vi "Spectrometer_R&S_2017.04.10.vi"(11 "position_xyz":T2 {"Position Z" min=0.0 max=10.0 step=0.001 format="%.3f"; "Position Y" min=-10.0 max=10.0 step=0.1 format="%.3f"; "Position X" min=-10.0 max=10.0 step=0.1 format="%.3f"}) -> ()   [LabVIEW 2014]
uses:
  <vilib>/DAQmx/write.llb/DAQmx Write (Digital Bool 1Line 1Point).vi
  <vilib>/Analysis/baseanly.llb/Vector x A.vi
  GLOBAL_VAR.vi
  <vilib>/DAQmx/miscellaneous.llb/DAQmx Fill In Error Info.vi
  <vilib>/Analysis/Matrix/Numeric/Conversions/Array To Matrix - RA2.vi
  <vilib>/DAQmx/create/channels.llb/DAQmx Create Channel (CO-Pulse Generation-Ticks).vi
  <vilib>/DAQmx/create/channels.llb/DAQmx Create Channel (DO-Digital Output).vi
  <vilib>/DAQmx/configure/trigger.llb/DAQmx Start Trigger (Digital Edge).vi
  <resource>/objmgr/daqmx.rc
  <vilib>/Analysis/NI_AALBase.lvlib
  <vilib>/Analysis/Matrix/NI_Matrix.lvlib
  <instrlib>/Rohde&Schwarz RF Signal Generator/Rohde&Schwarz RF Signal Generator.lvlib
panel:
  in  "sweep_parameters":T1={"Repetitions"=1, "Power dBm"=5.999999061226845, "Freq Start [Hz]"=2800000000.0, "Freq Stop [Hz]"=3000000000.0, "Step size [Hz]"=2500000.0, "Dwell Time [ms]"=0.09999999974525053} {"Dwell Time [ms]" format="%.3f"; "Step size [Hz]" format="%.2p"; "Freq Stop [Hz]" format="%.2p"; "Freq Start [Hz]" format="%.2p"; "Power dBm" format="%.2f"; "Repetitions" min=1 max=1000 step=1}
  out "File name":string
  in  "Save":bool
  in  "Stop":bool
  in  "generator_enable":bool
  out "Run":i32=100
  out "Remain":i32
  out "Intensity Graph":ext[][](graph)
  out "Histogram":cluster{ext[], ext[]}[](graph)=[{[2700000000.0, 2702500000.0, 2705000000.0, 2707500000.0, 2710000000.0, 2712500000.0, 2715000000.0, 2717500000.0, 2720000000.0, 2722500000.0, 2725000000.0, 2727500000.0, 2730000000.0, 2732500000.0, 2735000000.0, 2737500000.0, 2740000000.0, 2742500000.0, 2745000000.0, 2747500000.0, 2750000000.0, 2752500000.0, 2755000000.0, 2757500000.0, 2760000000.0, 2762500000.0, 2765000000.0, 2767500000.0, 2770000000.0, 2772500000.0, 2775000000.0, 2777500000.0, 2780000000.0, 2782500000.0, 2785000000.0, 2787500000.0, 2790000000.0, 2792500000.0, 2795000000.0, 2797500000.0, 2800000000.0, 2802500000.0, 2805000000.0, 2807500000.0, 2810000000.0, 2812500000.0, 2815000000.0, 2817500000.0, 2820000000.0, 2822500000.0, 2825000000.0, 2827500000.0, 2830000000.0, 2832500000.0, 2835000000.0, 2837500000.0, 2840000000.0, 2842500000.0, 2845000000.0, 2847500000.0, 2850000000.0, 2852500000.0, 2855000000.0, 2857500000.0, 2860000000.0, 2862500000.0, 2865000000.0, 2867500000.0, 2870000000.0, 2872500000.0, 2875000000.0, 2877500000.0, 2880000000.0, 2882500000.0, 2885000000.0, 2887500000.0, 2890000000.0, 2892500000.0, 2895000000.0, 2897500000.0, 2900000000.0, 2902500000.0, 2905000000.0, 2907500000.0, 2910000000.0, 2912500000.0, 2915000000.0, 2917500000.0, 2920000000.0, 2922500000.0, 2925000000.0, 2927500000.0, 2930000000.0, 2932500000.0, 2935000000.0, 2937500000.0, 2940000000.0, 2942500000.0, 2945000000.0, 2947500000.0, 2950000000.0, 2952500000.0, 2955000000.0, 2957500000.0, 2960000000.0, 2962500000.0, 2965000000.0, 2967500000.0, 2970000000.0, 2972500000.0, 2975000000.0, 2977500000.0, 2980000000.0, 2982500000.0, 2985000000.0, 2987500000.0, 2990000000.0, 2992500000.0, 2995000000.0, 2997500000.0, 3000000000.0], [26841.121559672197128, 27464.174520667373477, 27576.32405364650522, 29408.099758972323686, 27638.629349746022854, 27576.32405364650522, 27638.629349746022854, 27651.09040896592638, 28398.753962160138, 28311.526547620813311, 28236.76019230139215, 27912.772652583900449, 27850.467356484382814, 27875.389474924189868, 28174.454896201874515, 28697.819383437822648, 28685.35832421791912, 28535.825613579076798, 28809.968916416954391, 29046.729041595121403, 28647.975146558208541, 28523.36455435917327, 28062.305363222742772, 28174.454896201874515, 28473.520317479559163, 27738.31782350525107, 28423.676080599945054, 29133.956456134446093, 28859.8131532965685, 27638.629349746022854, 29133.956456134446093, 27763.239941945058124, 27352.024987688241733, 27439.252402227566423, 28822.429975636857918, 27526.479816766891112, 28548.286672798980325, 27838.006297264479286, 28847.352094076664972, 28884.735271736375553, 29271.02810755338489, 28884.735271736375553, 27289.7196915887241, 28971.962686275700243, 28336.448666060620365, 28548.286672798980325, 27975.077948683418082, 27763.239941945058124, 29470.405055071841321, 28822.429975636857918, 28087.227481662549826, 28286.604429181006259, 27352.024987688241733, 27401.869224567855841, 28398.753962160138, 29308.411285213095471, 28485.98137669946269, 28585.669850458690906, 28710.280442657726175, 28236.76019230139215, 28311.526547620813311, 27576.32405364650522, 27302.180750808627625, 28299.065488400909786, 26878.504737331907709, 28809.968916416954391, 29420.560818192227213, 28859.8131532965685, 27750.778882725154597, 28535.825613579076798, 28398.753962160138, 28261.682310741199204, 28947.040567835893189, 28361.370784500427419, 28785.046797977147337, 28610.59196889849796, 27476.635579887277004, 28062.305363222742772, 28311.526547620813311, 28809.968916416954391, 28647.975146558208541, 28112.14960010235688, 28822.429975636857918, 27738.31782350525107, 28199.377014641681569, 28510.903495139269744, 27451.71346144746995, 28074.766422442646299, 27725.856764285347543, 28635.514087338305014, 28834.891034856761445, 27376.947106128048787, 29096.573278474735512, 28274.143369961102731, 29034.267982375217876, 28560.747732018883852, 27277.258632368820573, 28884.735271736375553, 28049.844304002839245, 27975.077948683418082, 26965.732151871232396, 28809.968916416954391, 28000.000067123225136, 27127.725921729978248, 28037.383244782935718, 28000.000067123225136, 27277.258632368820573, 27800.623119604768705, 28087.227481662549826, 27501.557698327084058, 26778.816263572679492, 26429.906605415380737, 27526.479816766891112, 26442.367664635284264, 26479.750842294994845, 27775.701001164961651, 27040.498507190653559, 26429.906605415380737, 27750.778882725154597, 27464.174520667373477, 27925.233711803803976]}, {[2700000000.0, 2702500000.0, 2705000000.0, 2707500000.0, 2710000000.0, 2712500000.0, 2715000000.0, 2717500000.0, 2720000000.0, 2722500000.0, 2725000000.0, 2727500000.0, 2730000000.0, 2732500000.0, 2735000000.0, 2737500000.0, 2740000000.0, 2742500000.0, 2745000000.0, 2747500000.0, 2750000000.0, 2752500000.0, 2755000000.0, 2757500000.0, 2760000000.0, 2762500000.0, 2765000000.0, 2767500000.0, 2770000000.0, 2772500000.0, 2775000000.0, 2777500000.0, 2780000000.0, 2782500000.0, 2785000000.0, 2787500000.0, 2790000000.0, 2792500000.0, 2795000000.0, 2797500000.0, 2800000000.0, 2802500000.0, 2805000000.0, 2807500000.0, 2810000000.0, 2812500000.0, 2815000000.0, 2817500000.0, 2820000000.0, 2822500000.0, 2825000000.0, 2827500000.0, 2830000000.0, 2832500000.0, 2835000000.0, 2837500000.0, 2840000000.0, 2842500000.0, 2845000000.0, 2847500000.0, 2850000000.0, 2852500000.0, 2855000000.0, 2857500000.0, 2860000000.0, 2862500000.0, 2865000000.0, 2867500000.0, 2870000000.0, 2872500000.0, 2875000000.0, 2877500000.0, 2880000000.0, 2882500000.0, 2885000000.0, 2887500000.0, 2890000000.0, 2892500000.0, 2895000000.0, 2897500000.0, 2900000000.0, 2902500000.0, 2905000000.0, 2907500000.0, 2910000000.0, 2912500000.0, 2915000000.0, 2917500000.0, 2920000000.0, 2922500000.0, 2925000000.0, 2927500000.0, 2930000000.0, 2932500000.0, 2935000000.0, 2937500000.0, 2940000000.0, 2942500000.0, 2945000000.0, 2947500000.0, 2950000000.0, 2952500000.0, 2955000000.0, 2957500000.0, 2960000000.0, 2962500000.0, 2965000000.0, 2967500000.0, 2970000000.0, 2972500000.0, 2975000000.0, 2977500000.0, 2980000000.0, 2982500000.0, 2985000000.0, 2987500000.0, 2990000000.0, 2992500000.0, 2995000000.0, 2997500000.0, 3000000000.0], [27662.305362263847, 27614.704116043806, 27558.75396014644, 27479.62623410005, 27635.264863756656, 27635.514084941045, 27523.73838373851, 27614.704116043802, 27583.17763621744, 27571.58885114293, 27593.520315369973, 27605.109100444486, 27505.545237277456, 27540.685424277577, 27573.831841802512, 27521.74461426332, 27747.788228512374, 27553.395704681883, 27408.099754177805, 27507.040564383846, 27553.769536458476, 27450.09352374888, 27547.16517507192, 27590.529661157172, 27485.98137430221, 27331.838071751987, 27460.06237112481, 27420.436202805507, 27402.99071989765, 27434.64181031619, 27576.697885423117, 27476.38635870286, 27470.654271461714, 27460.311592309215, 27451.962682631867, 27448.722807234688, 27469.781997316335, 27462.056140599987, 27364.23682572375, 27414.081062603364, 27456.573274543232, 27499.688539444087, 27488.598196738385, 27439.252402227583, 27451.215019078678, 27574.45489476352, 27513.894146954794, 27562.741499096825, 27559.377013107456, 27384.42374165998, 27576.074832462113, 27480.747729429848, 27504.423741947663, 27448.099754273695, 27508.90972326683, 27439.50162341197, 27397.383243248685, 27424.54835234809, 27331.21501879102, 27477.258632848276, 27459.68853934821, 27434.267978539607, 27381.05925567063, 27417.07171681613, 27347.912838145676, 27456.82249572762, 27392.398819560723, 27427.539006560855, 27402.86610930546, 27384.79757343659, 27482.86610949723, 27504.049910171063, 27508.037449121424, 27430.778881958024, 27495.202558124915, 27442.367667032533, 27426.16829004667, 27367.60131171313, 27402.616888121054, 27600.00006616432, 27539.68853953999, 27533.58262052224, 27462.305361784383, 27564.361436795392, 27572.087293511737, 27503.55146780227, 27476.137137518494, 27474.766421004293, 27580.560813781274, 27579.813150228085, 27592.024988263576, 27505.296016093063, 27570.84118758975, 27614.953337228195, 27611.215019462234, 27484.236826011424, 27503.925299578863, 27544.54835263575, 27602.616888600503, 27550.903492837893, 27593.769536554377, 27516.63557998317, 27611.962683015438, 27551.028103430108, 27655.701000877292, 27659.688539827646, 27578.5670443061, 27729.59508205134, 27610.093524132444, 27489.968913252564, 27615.202558412602, 27486.479816671, 27421.059255766515, 27418.56704392252, 27449.221249603488, 27600.996950901917, 27543.92529967475, 27425.17140530909, 27466.04367955036, 27523.987604922913, 27501.183866550484]}]
  in  "start":bool
  in  "stop":bool
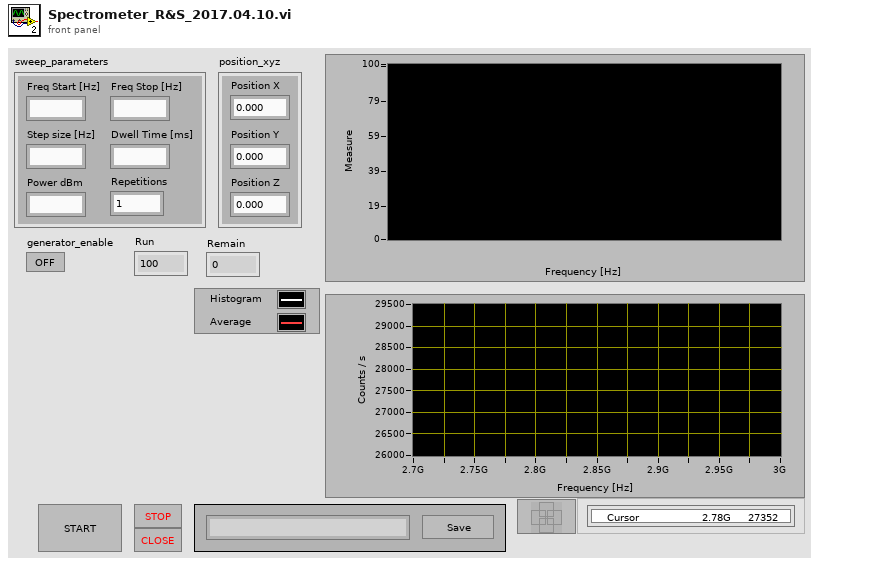
[diagram p1: front panel]
types:
  T1 = cluster{"Repetitions":i32, "Power dBm":ext, "Freq Start [Hz]":ext, "Freq Stop [Hz]":ext, "Step size [Hz]":ext, "Dwell Time [ms]":ext}
  T2 = cluster{"Position X":dbl, "Position Y":dbl, "Position Z":dbl}
  T3 = enum16{"stand-by", "init", "config", "acquisition", "processing", "close", "Set Variables"}
  T4 = typedef "NI_Matrix.lvlib/RealMatrix.ctl" = dbl[][]
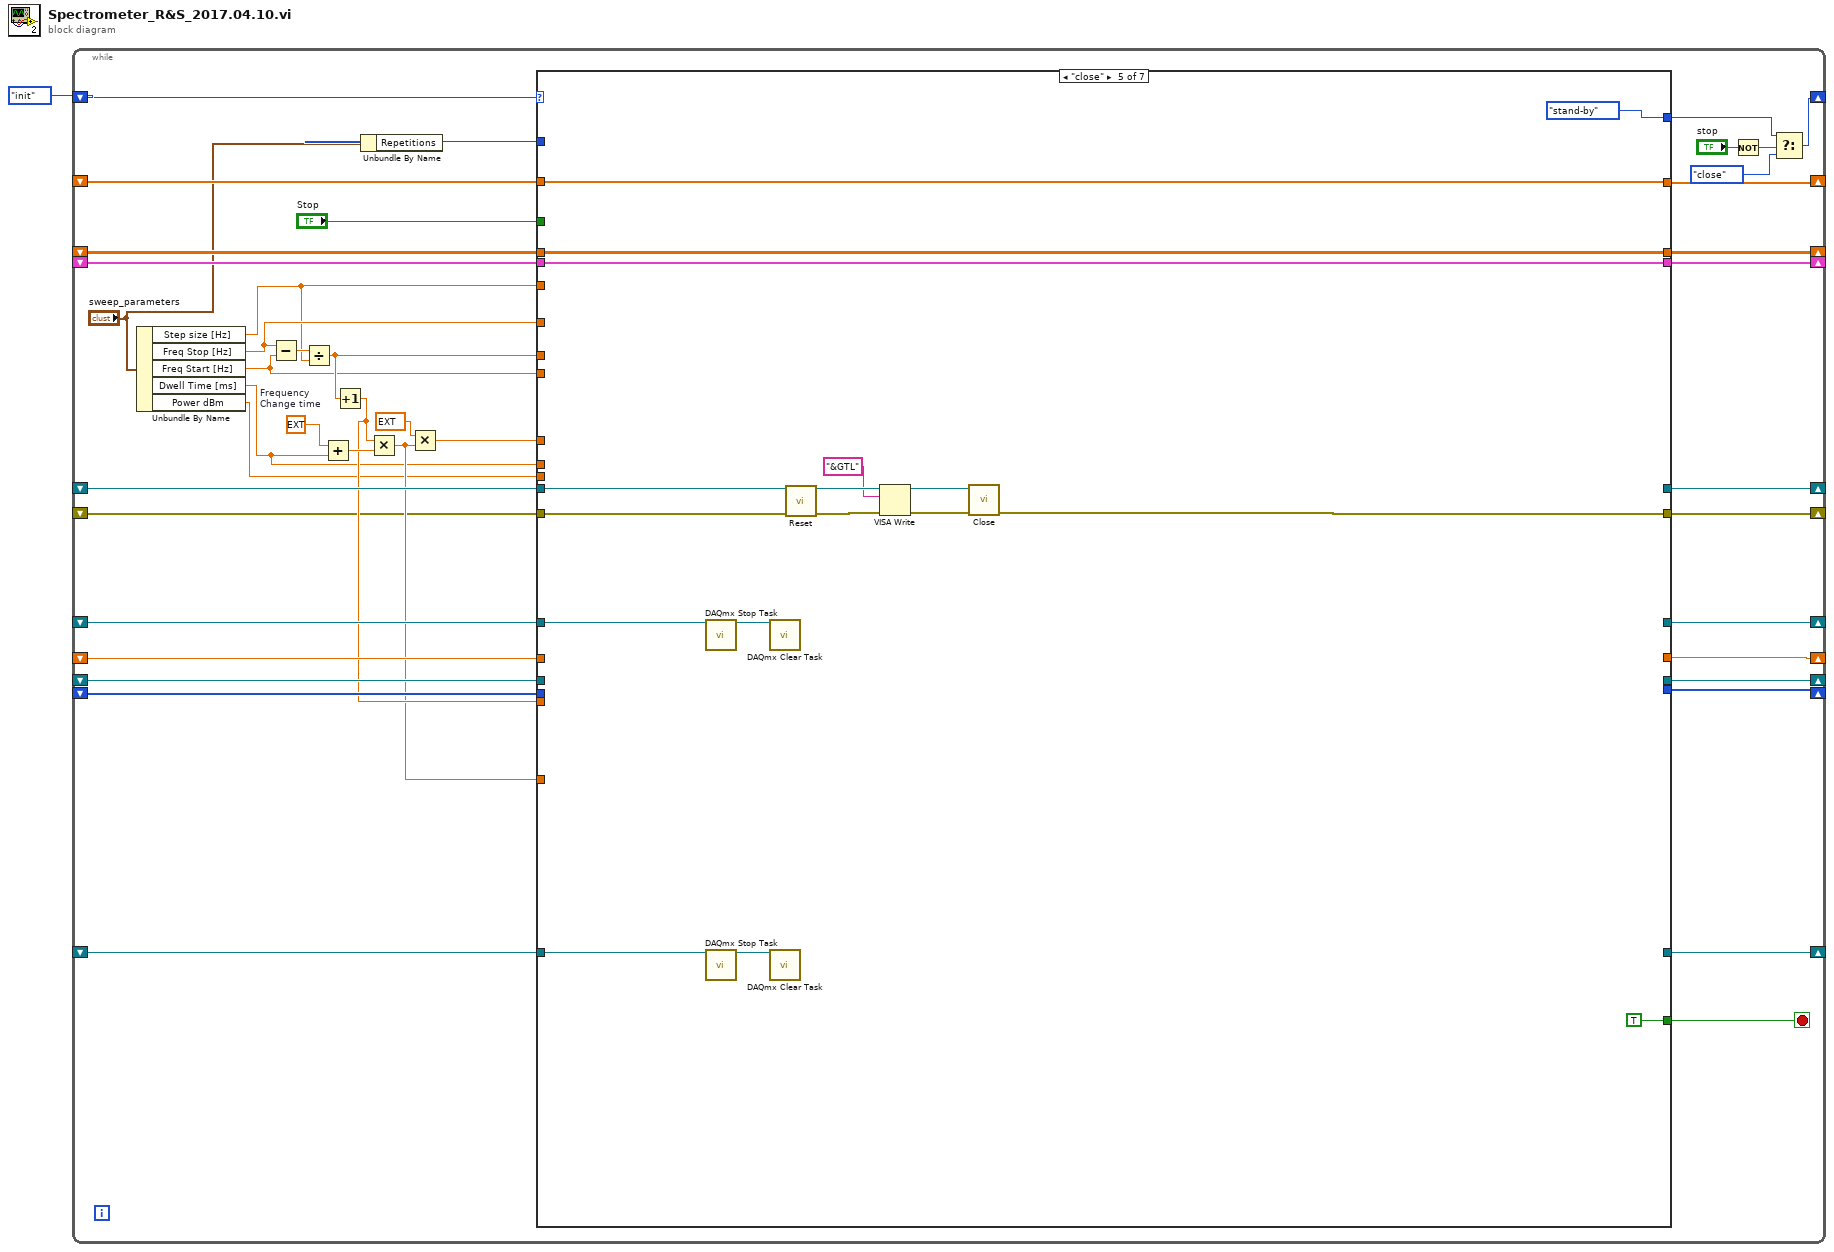
[diagram p0: block diagram]
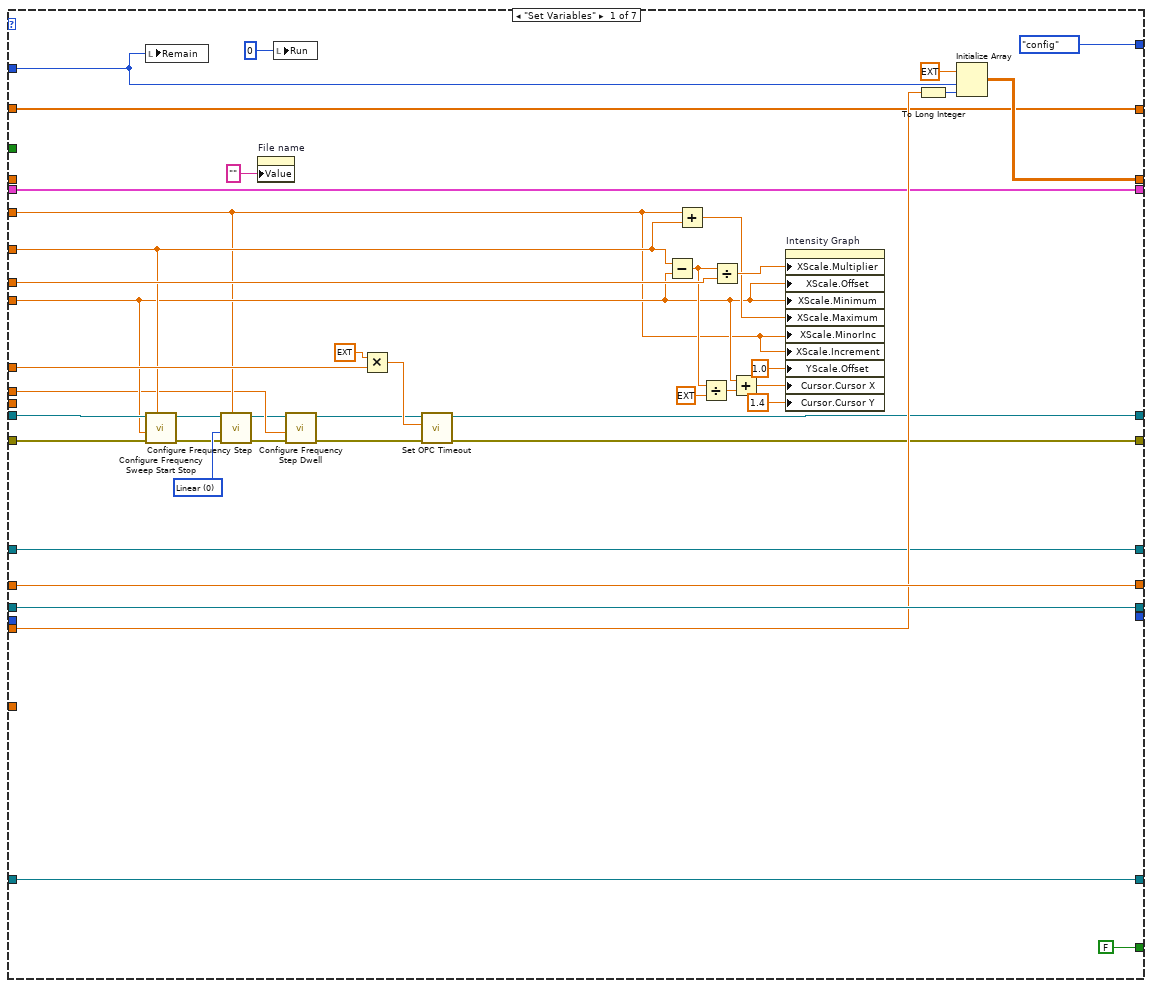
[diagram p2: hidden frame]
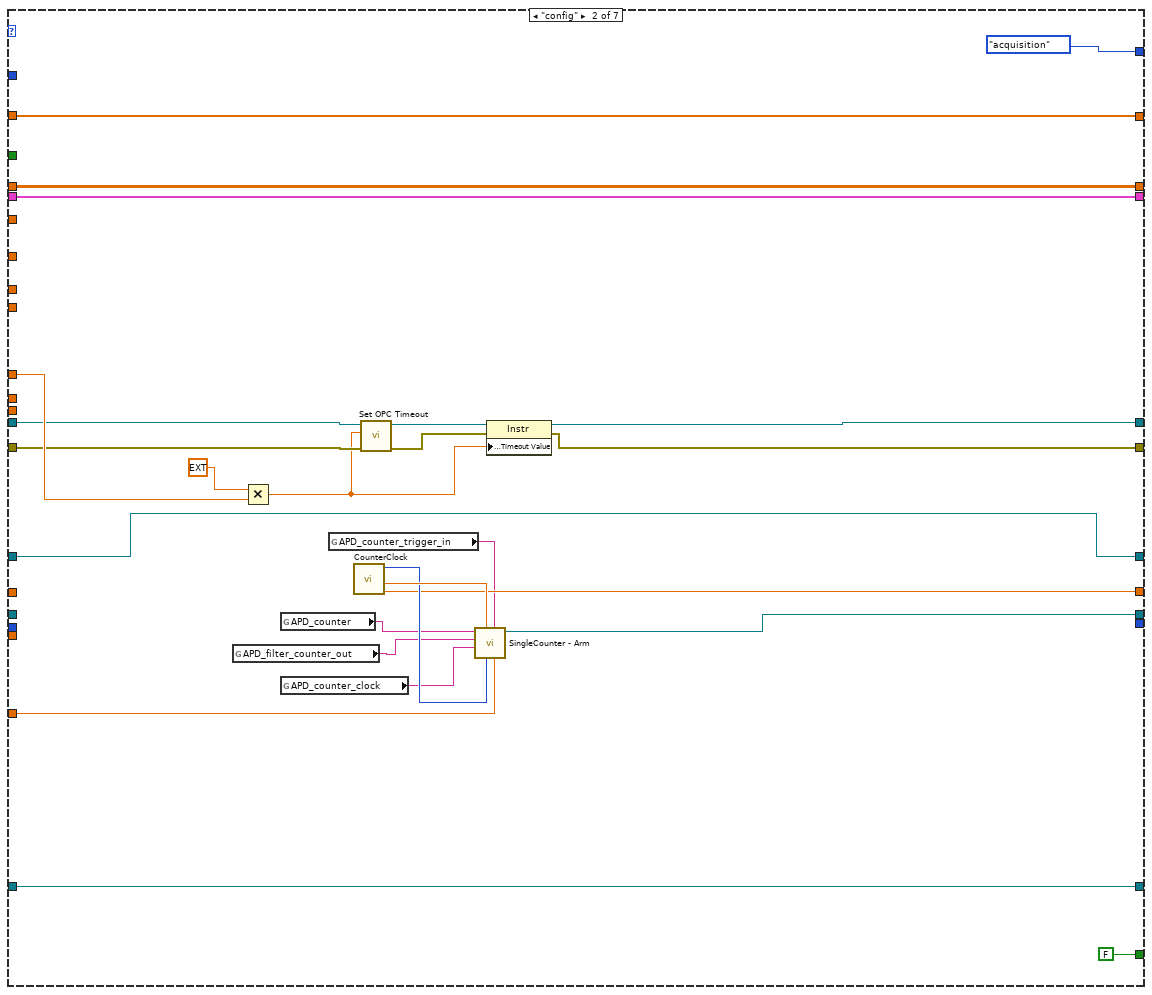
[diagram p3: hidden frame]
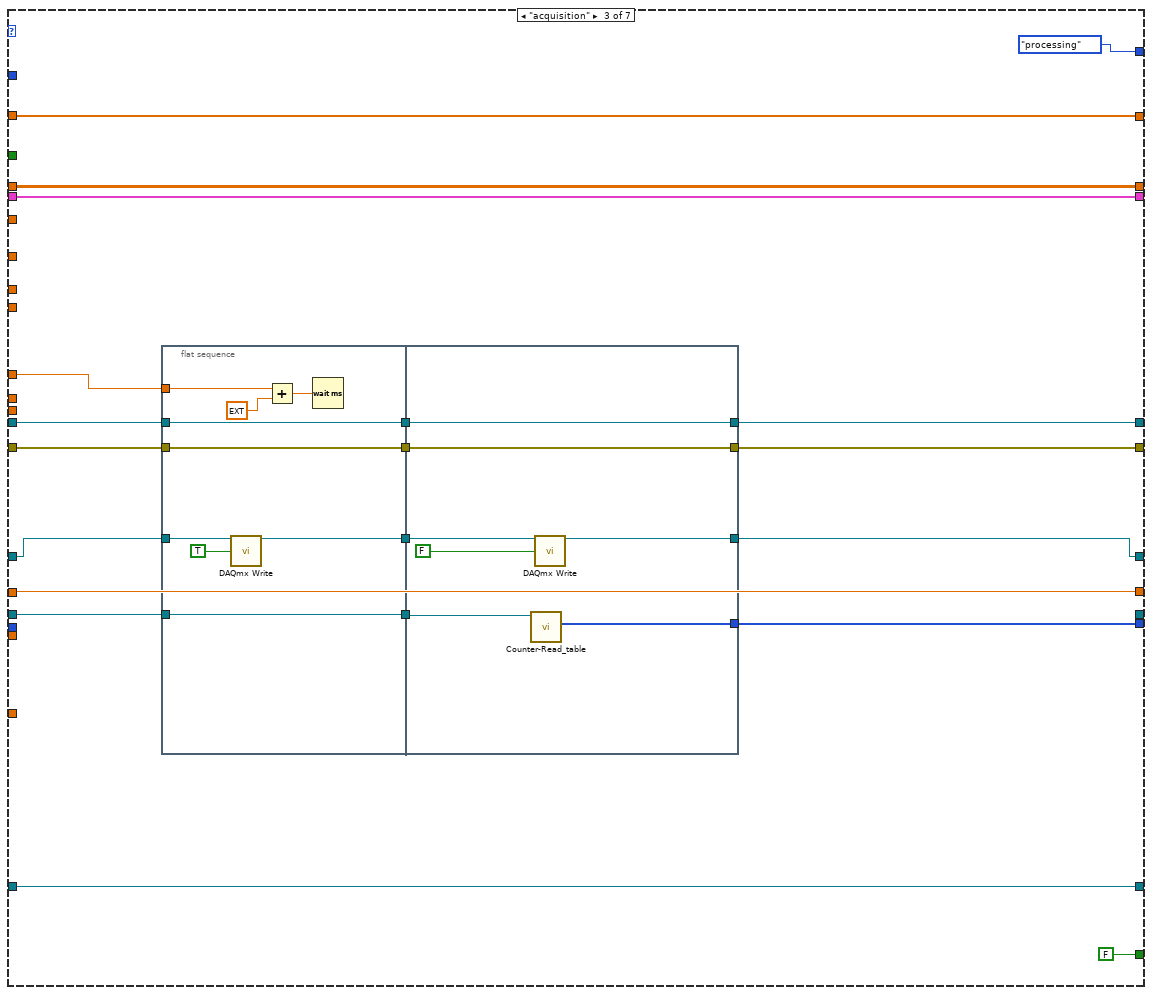
[diagram p4: hidden frame]
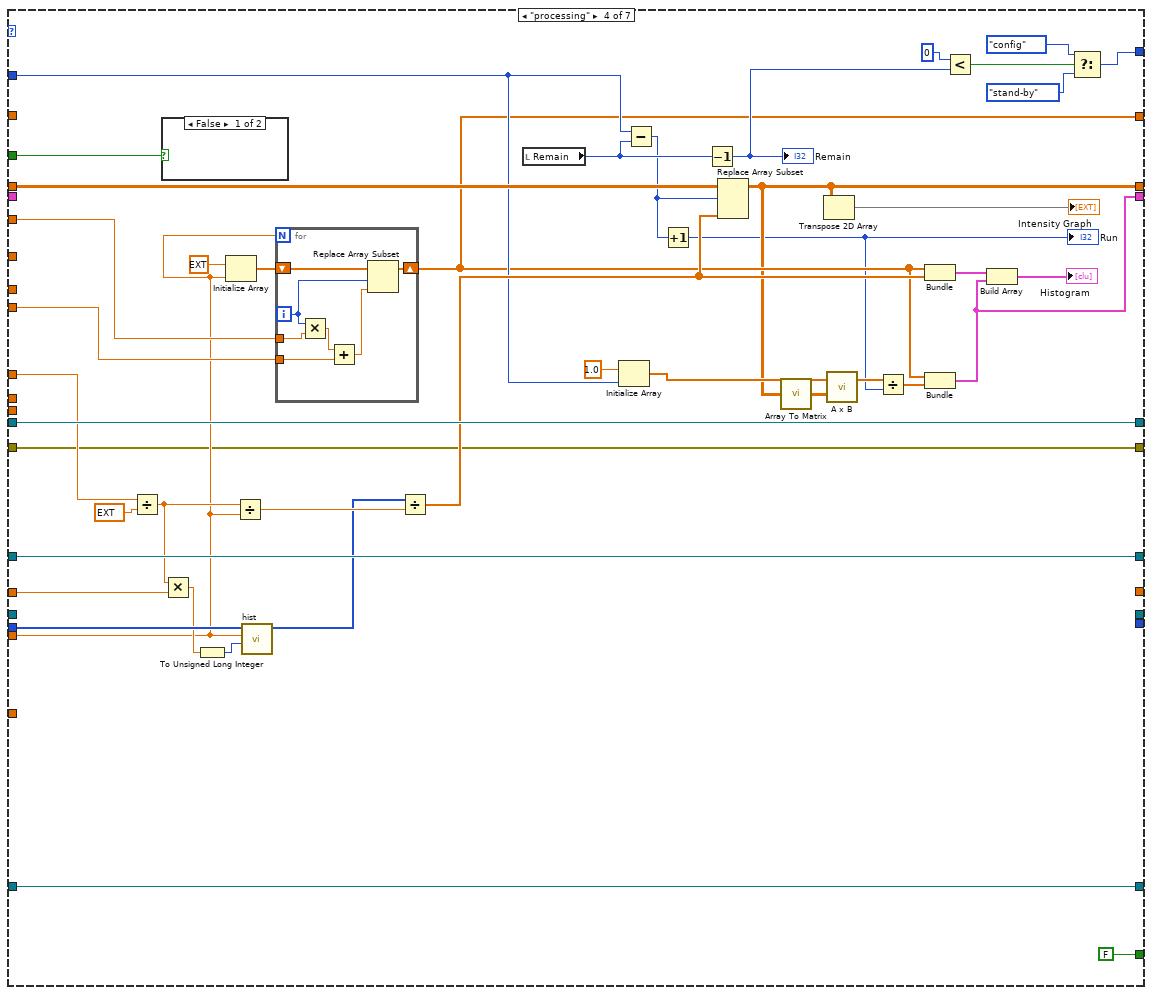
[diagram p5: hidden frame]
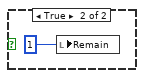
[diagram p6: hidden frame]
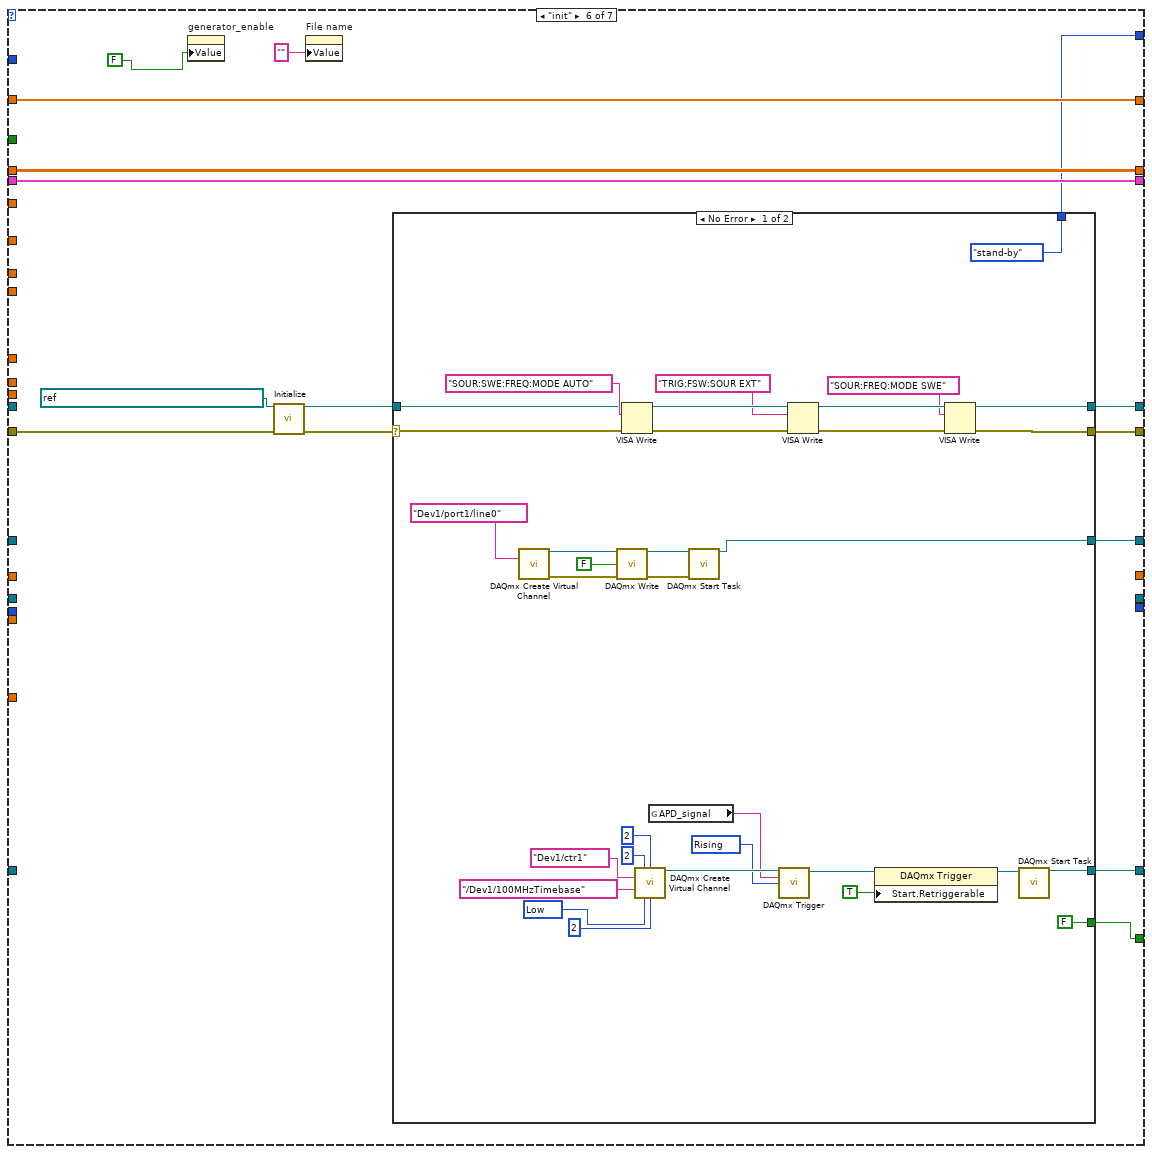
[diagram p7: hidden frame]
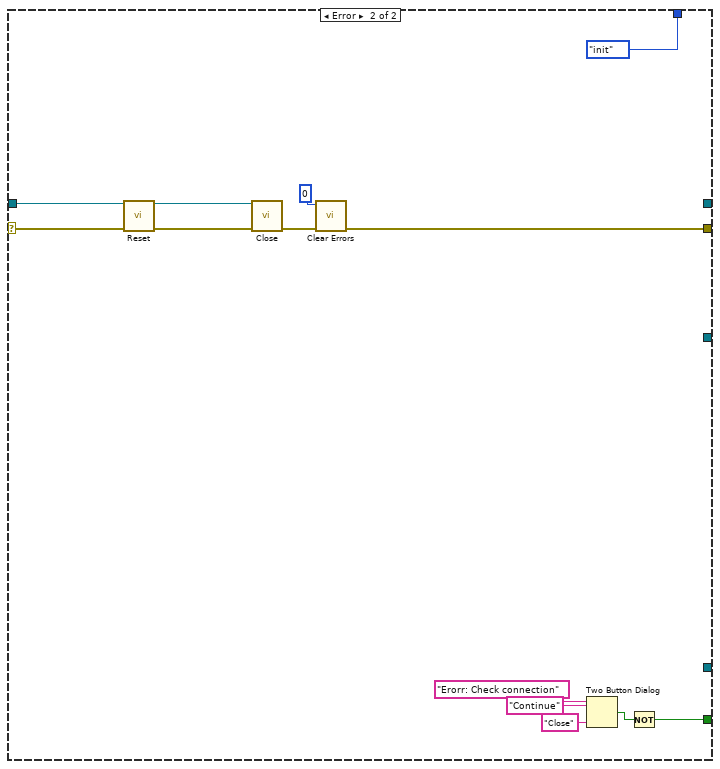
[diagram p8: hidden frame]
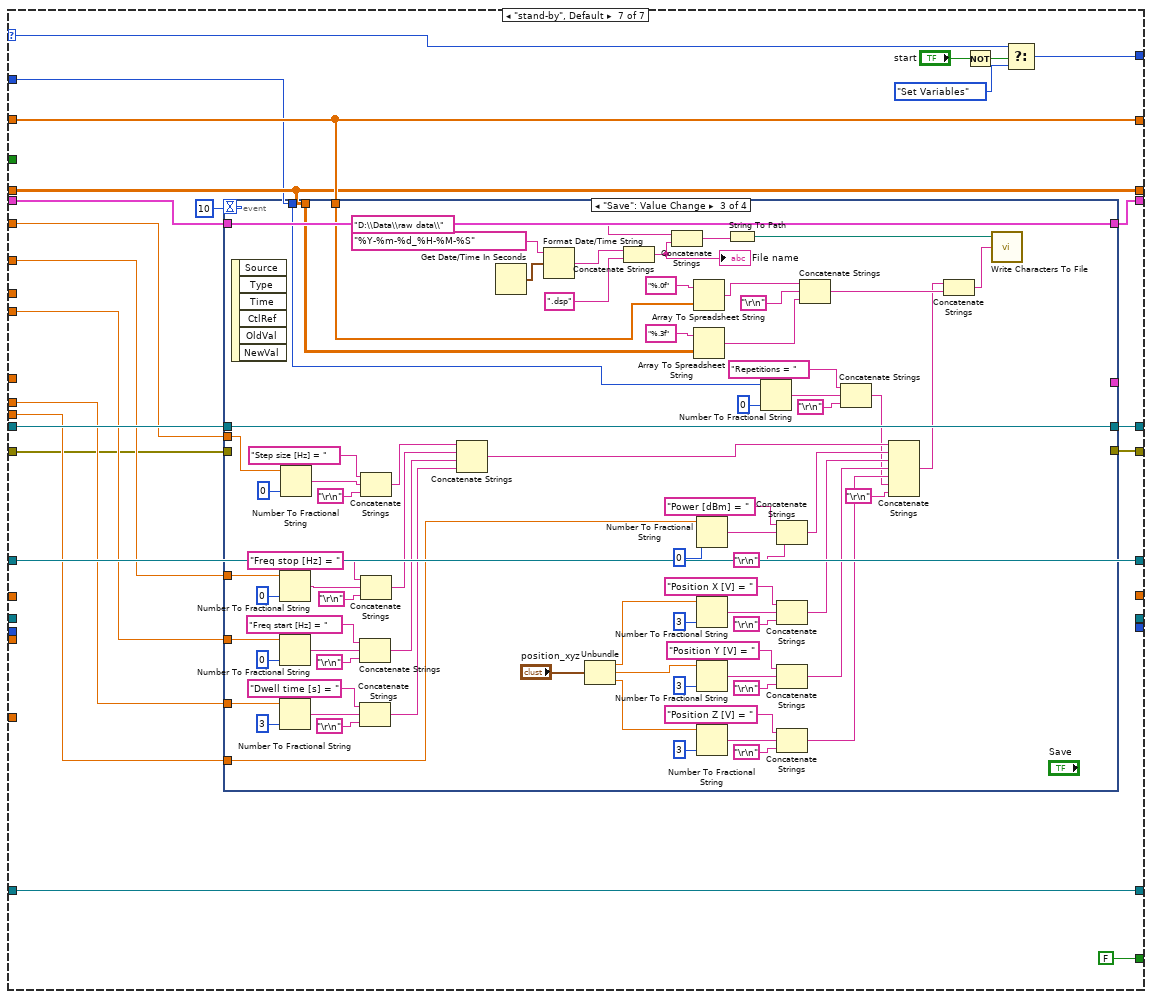
[diagram p9: hidden frame]
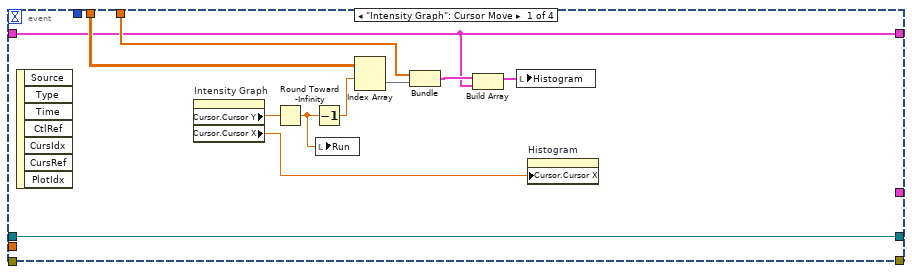
[diagram p10: hidden frame]
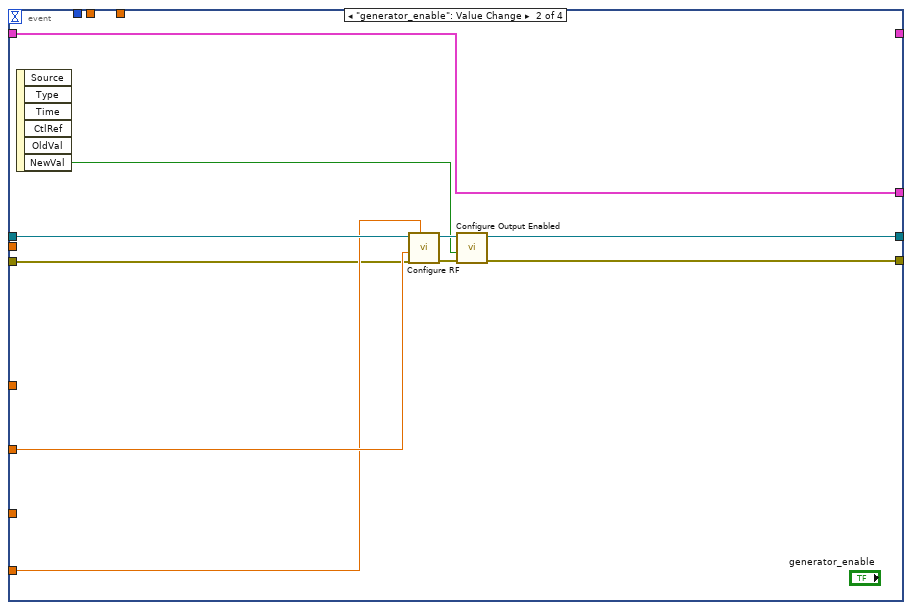
[diagram p11: hidden frame]
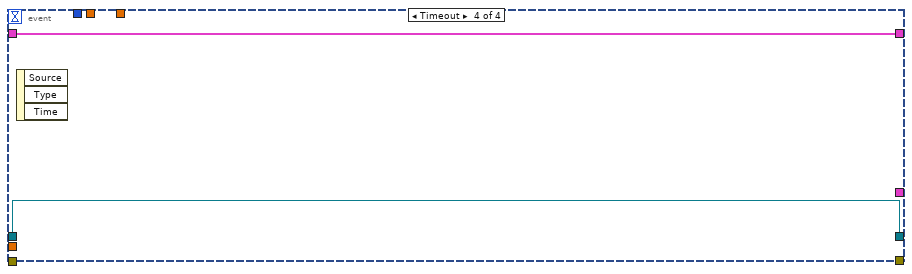
[diagram p12: hidden frame]
diagram:
  n1 = while {
    shift-right: [w30] -> _
    shift-left: T3."init" -> [w44]
    shift-right: [w40] -> _
    shift-left: _ -> [w39]
    shift-right: [w12] -> _
    shift-left: _ -> [w38]
    shift-right: [w37] -> _
    shift-left: _ -> [w36]
    shift-right: [w35] -> _
    shift-left: _ -> [w34]
    shift-right: [w28] -> _
    shift-left: _ -> [w27]
    shift-right: [w21] -> _
    shift-left: _ -> [w23]
    shift-right: [w20] -> _
    shift-left: _ -> [w19]
    shift-right: [w17] -> _
    shift-left: _ -> [w16]
    shift-right: [w15] -> _
    shift-left: _ -> [w14]
    shift-right: [w11] -> _
    shift-left: _ -> [w10]
    stop <- w29 stop-if-true
    w9 = ext 0.0  # Frequency Change time
    n2 = Unbundle By Name("sweep_parameters") -> ("Step size [Hz]"=w4:ext, "Freq Stop [Hz]"=w5:ext, "Freq Start [Hz]"=w3:ext, "Dwell Time [ms]"=w6:ext, "Power dBm"=w7:ext)
    n3 = Subtract(x=w5, y=w3) -> (x-y=w43:ext)
    n4 = Divide(x=w43, y=w4) -> (x/y=w24:ext)
    n5 = Add(x=w9, y=w6) -> (x+y=w42:ext)
    n6 = Increment(x=w24) -> (x+1=w25:ext)
    n7 = Unbundle By Name("sweep_parameters") -> ("Repetitions"=w8:i32)
    n8 = Multiply(x=w25, y=w42) -> (x*y=w18:ext)
    n9 = Multiply(x=ext 1000.0 ("y"), y=w18) -> (x*y=w41:ext)
    n10 = case shown="\"close\"" w44 {
      selector: w44 -> [_ _ _ _ _ _ w299]
      tunnel: [T3."config" T3."acquisition" T3."processing" w176 T3."stand-by" w221 w298] -> w31
      tunnel: [w46 w94 w130 w184 _ w223 w285] -> w40
      tunnel: [w61 w111 w117 w183 _ w222 w296] -> w12
      tunnel: w39 -> [w64 w97 w131 w184 w212 _ w286]
      tunnel: w38 -> [w61 w111 w118 w183 w215 _ w296]
      tunnel: w4 -> [w55 _ _ w182 _ _ w284]
      tunnel: w5 -> [w59 _ _ _ _ _ w283]
      tunnel: w3 -> [w58 _ _ w169 _ _ w282]
      tunnel: w41 -> [w62 w99 w116 w179 _ _ _]
      tunnel: w6 -> [w54 _ _ _ _ _ w281]
      tunnel: [w82 w107 _ _ _ _ _] -> w37
      tunnel: w36 -> [w82 _ w129 _ _ _ _]
      tunnel: [_ _ w128 _ _ _ _] -> w35
      tunnel: w34 -> [_ _ _ w189 _ _ _]
      tunnel: [FALSE FALSE FALSE FALSE TRUE w219 FALSE] -> w29
      tunnel: [w81 w106 w126 _ _ _ _] -> w28
      tunnel: w27 -> [w81 _ w126 w187 _ _ _]
      tunnel: w25 -> [w78 _ _ w164 _ _ _]
      tunnel: w24 -> [w77 _ _ _ _ _ _]
      tunnel: w7 -> [_ _ _ _ _ _ w280]
      tunnel: w8 -> [w68 _ _ w161 _ _ w279]
      tunnel: w23 -> [_ w105 w125 w173 w211 w230 w290]
      tunnel: [w80 w105 w125 w153 w211 w230 w290] -> w21
      tunnel: [w69 w103 w123 w159 w209 w229 w292] -> w20
      tunnel: w19 -> [w69 w103 w123 _ w209 w229 w292]
      tunnel: w18 -> [_ w102 _ _ _ _ _]
      tunnel: [w66 w101 w122 w166 _ w220 w289] -> w17
      tunnel: w16 -> [w66 w101 w122 w166 w207 _ w289]
      tunnel: [w65 w100 w121 w151 w206 w228 w287] -> w15
      tunnel: w14 -> [w65 w100 w121 _ w206 w228 w288]
      tunnel: "Stop" -> [_ _ _ w154 _ _ _]
      tunnel: [w45 w91 w119 w152 w204 w218 w277] -> w11
      tunnel: w10 -> [w56 w96 w120 w152 w205 w217 w278]
      frame "Set Variables" {
        w53 = 0 items=["Linear", "Logarithmic"] ("Scaling (Linear)")
        n11 = local write "Remain"(w68) -> ()
        n12 = call <instrlib>:"Configure Frequency Sweep Start Stop.vi"("Stop (500.0e6)"=w59, "error in (no error)"=w56, "Start (100.0e6)"=w58, "VISA resource name"=w64) -> ("error out"=w51:errorcluster, "VISA resource name out"=w52:refnum<visa-resource-name>)  [unwired: 6 in]
        n13 = call <instrlib>:"Configure Frequency Step.vi"("Step Size (100.0e3)"=w55, "error in (no error)"=w51, "Scaling (Linear)"=w53, "VISA resource name"=w52) -> ("error out"=w49:errorcluster, "VISA resource name out"=w50:refnum<visa-resource-name>)  [unwired: 6 in]
        n14 = property on="File name" class="Str"("Value"="" ("File name")) -> ()  [unwired: 2 in, 2 out]
        n15 = local write "Run"(0 ("Run")) -> ()
        n16 = call <instrlib>:"Configure Frequency Step Dwell.vi"("error in (no error)"=w49, "Dwell (10.0e-3)"=w54, "VISA resource name"=w50) -> ("error out"=w47:errorcluster, "VISA resource name out"=w48:refnum<visa-resource-name>)  [unwired: 7 in]
        n17 = Multiply(x=ext 1.100000023841858, y=w62) -> (x*y=w57:ext)
        n18 = call <instrlib>:"Set OPC Timeout.vi"("error in (no error)"=w47, "OPC Timeout (0)"=w57, "VISA resource name"=w48) -> ("error out"=w45:errorcluster, "VISA resource name out"=w46:refnum<visa-resource-name>)  [unwired: 7 in]
        n19 = Subtract(x=w59, y=w58) -> (x-y=w74:ext)
        n20 = Add(x=w55, y=w59) -> (x+y=w76:ext)
        n21 = Divide(x=w74, y=ext 2.0) -> (x/y=w70:ext)
        n22 = Divide(x=w74, y=w77) -> (x/y=w79:ext)
        n23 = Add(x=w58, y=w70) -> (x+y=w71:ext)
        n24 = property on="Intensity Graph" class="IntGraph (strict)"("XScale.Multiplier"=w79, "XScale.Offset"=w58, "XScale.Minimum"=w58, "XScale.Maximum"=w76, "XScale.MinorInc"=w55, "XScale.Increment"=w55, "YScale.Offset"=1.0 ("Y Scale.Offset and Multiplier:Offset"), "Cursor.Cursor X"=w71, "Cursor.Cursor Y"=1.4 ("Cursor.Cursor Position:Cursor Y")) -> ()  [unwired: 2 in, 2 out]
        n25 = To Long Integer(number=w78) -> (32bit integer=w84:i32)
        n26 = Initialize Array(ext 0.0 ("element"), w68, w84) -> (w80:ext[][])
      }
      frame "config" {
        n27 = global read "GLOBAL_VAR.vi" "APD_filter_counter_out"() -> (w87:tag)
        n28 = Multiply(x=ext 5.0 ("lower limit"), y=w99) -> (x*y=w93:ext)
        n29 = global read "GLOBAL_VAR.vi" "APD_counter"() -> (w89:tag)
        n30 = global read "GLOBAL_VAR.vi" "APD_counter_clock"() -> (w88:tag)
        n31 = global read "GLOBAL_VAR.vi" "APD_counter_trigger_in"() -> (w90:tag)
        n32 = call "CounterClock.vi"() -> ("Counter clock rate divided by prescaler"=w106:dbl, "Counter clock rate"=w109:dbl, "CI.Prescaler"=w108:u32)  [unwired: 8 in, 1 out]
        n33 = call <instrlib>:"Set OPC Timeout.vi"("error in (no error)"=w96, "OPC Timeout (0)"=w93, "VISA resource name"=w97) -> ("error out"=w92:errorcluster, "VISA resource name out"=w95:refnum<visa-resource-name>)  [unwired: 7 in]
        n34 = call "SingleCounter - Arm.vi"("Duration"=w102, "Trigger Source"=w90, "CI.Prescaler"=w108, "Sampling Rate"=w109, "Clock Source"=w88, "External Timing Source"=w87, "counter"=w89) -> ("task out"=w107:refnum<k21>)  [unwired: 3 in, 1 out]
        n35 = property class="Instr"(reference=w95, error in=w92, "General Settings:Timeout Value"=w93) -> (reference out=w94:refnum<visa-resource-name>, error out=w91:errorcluster)
      }
      frame "acquisition" {
        n36 = flat-sequence {
          tunnel: w131 -> [w136]
          tunnel: [w139] -> w115
          tunnel: [w138] -> w114
          tunnel: w129 -> [w138]
          tunnel: w120 -> [w135]
          tunnel: w118 -> [w137]
          tunnel: w116 -> [w133]
          tunnel: [w136] -> w113
          tunnel: [w135] -> w112
          tunnel: [w143] -> w117
          tunnel: [w142] -> w130
          tunnel: w115 -> [w146]
          tunnel: w114 -> [w144]
          tunnel: [w145] -> w128
          tunnel: [w141] -> w119
          tunnel: w113 -> [w142]
          tunnel: w112 -> [w141]
          frame #0 {
            n37 = call-poly <vilib>:"DAQmx Write.vi"("task/channels in"=w137, "data"=TRUE) -> ("task out"=w139:refnum<k21>)  [unwired: 11 in, 2 out]
            n38 = Add(x=w133, y=ext 1.1) -> (x+y=w134:ext)
            n39 = Wait (ms)(milliseconds to wait=w134) -> ()  [unwired: 1 out]
          }
          frame #1 {
            n40 = call "Counter-Read_table.vi"("task in"=w144) -> ("time tags"=w145:u32[])  [unwired: 9 in, 1 out]
            n41 = call-poly <vilib>:"DAQmx Write.vi"("task/channels in"=w146, "data"=FALSE) -> ("task out"=w143:refnum<k21>)  [unwired: 11 in, 2 out]
          }
        }
      }
      frame "processing" {
        n42 = Divide(x=w179, y=ext 1000.0) -> (x/y=w178:ext)
        n43 = case shown="False" w154 {
          frame False {
          }
          frame True {
            n44 = local write "Remain"(1) -> ()
          }
        }
        n45 = Multiply(x=w178, y=w187) -> (x*y=w185:ext)
        n46 = To Unsigned Long Integer(number=w185) -> (unsigned 32bit integer=w186:u32)
        n47 = Initialize Array(ext 0.0 ("element"), w164) -> (w180:ext[])
        n48 = Divide(x=w178, y=w164) -> (x/y=w177:ext)
        n49 = call "hist.vi"("#clock cycles"=w186, "#bins"=w164, "counter timetag list"=w189) -> ("histogram"=w150:i32[])  [unwired: 7 in]
        n50 = for {
          N: w164 -> [_]
          tunnel: w182 -> [w194]
          shift-right: [w198] -> w159
          shift-left: w180 -> [w197]
          tunnel: w169 -> [w196]
          i -> [w195]
          n51 = Multiply(x=w195, y=w194) -> (x*y=w193:ext)
          n52 = Add(x=w193, y=w196) -> (x+y=w192:ext)
          n53 = Replace Array Subset(array=w197, new element=w192, index=w195) -> (w198:ext[])
        }
        n54 = Divide(x=w150, y=w177) -> (x/y=w165:ext[])
        n55 = local read "Remain"() -> (w168:i32)
        n56 = Initialize Array(1.0 ("element"), w161) -> (w160:dbl[])
        n57 = Subtract(x=w161, y=w168) -> (x-y=w167:i32)
        n58 = Increment(x=w167) -> (x+1=w148:i32)
        "Run" <- w148
        n59 = Decrement(x=w168) -> (x-1=w170:i32)
        "Remain" <- w170
        n60 = Replace Array Subset(array=w173, new element=w165, index (row)=w167) -> (w153:ext[][])  [unwired: 1 in]
        n61 = call-poly <vilib>:"Array To Matrix.vi"("Real 2D Array"=w153) -> ("Real Matrix"=w163:T4)
        n62 = Transpose 2D Array(2D array=w153) -> (transposed array=→"Intensity Graph":ext[][])
        n63 = call-poly <vilib>:"A x B.vi"("Matrix A"=w163, "Vector V'"=w160) -> ("V' x A"=w157:dbl[])  [unwired: 1 out]
        n64 = Divide(x=w157, y=w148) -> (x/y=w158:dbl[])
        n65 = Bundle(w159, w165) -> (w156:cluster{ext[], ext[]})  [unwired: 1 in]
        n66 = Bundle(w159, w158) -> (w151:cluster{ext[], dbl[]})  [unwired: 1 in]
        n67 = Less?(x=0, y=w170) -> (x < y?=w174:bool)
        n68 = Build Array(w156, w151) -> (→"Histogram":cluster{ext[], ext[]}[])
        n69 = Select(t=T3."config", s=w174, f=T3."stand-by") -> (s? t:f=w176:T3)
      }
      frame "close" {
        n70 = call <vilib>:"DAQmx Stop Task.vi"("task/channels in"=w215) -> ("task out"=w214:refnum<k21>)  [unwired: 13 in, 1 out]
        n71 = call <vilib>:"DAQmx Stop Task.vi"("task/channels in"=w207) -> ("task out"=w208:refnum<k21>)  [unwired: 13 in, 1 out]
        n72 = call <vilib>:"DAQmx Clear Task.vi"("task in"=w214) -> ()  [unwired: 14 in, 1 out]
        n73 = call <vilib>:"DAQmx Clear Task.vi"("task in"=w208) -> ()  [unwired: 14 in, 1 out]
        n74 = call <instrlib>:"Reset.vi"("VISA resource name"=w212, "error in (no error)"=w205) -> ("VISA resource name out"=w203:refnum<visa-resource-name>, "error out"=w201:errorcluster)  [unwired: 12 in]
        n75 = VISA Write(VISA resource name=w203, write buffer="&GTL", error in (no error)=w201) -> (VISA resource name out=w202:refnum<visa-resource-name>, error out=w200:errorcluster)  [unwired: 1 out]
        n76 = call <instrlib>:"Close.vi"("error in (no error)"=w200, "VISA resource name"=w202) -> ("error out"=w204:errorcluster)  [unwired: 9 in]
      }
      frame "init" {
        n77 = property on="generator_enable" class="Bool (strict)"("Value"=FALSE ("Generator  output")) -> ()  [unwired: 2 in, 2 out]
        n78 = call <instrlib>:"Initialize.vi"("VISA resource name"=refnum<visa-resource-name> "USB0::0x0AAD::0x005F::262159::INSTR", "error in (no error)"=w217) -> ("VISA resource name out"=w224:refnum<visa-resource-name>, "error out"=w225:errorcluster)  [unwired: 12 in]
        n79 = property on="File name" class="Str"("Value"="" ("File name")) -> ()  [unwired: 2 in, 2 out]
        n80 = case shown="No Error" w225 {
          selector: w225 -> [w242 w275]
          tunnel: [w240 _] -> w223
          tunnel: w224 -> [w239 w276]
          tunnel: [w232 _] -> w222
          tunnel: [T3."stand-by" T3."init"] -> w221
          tunnel: [w251 _] -> w220
          tunnel: [FALSE w267] -> w219
          tunnel: [w241 w264] -> w218
          frame No Error {
            w257 = 10280 items=["Rising"=10280, "Falling"=10171] ("edge")
            w253 = 10214 items=["High"=10192, "Low"=10214] ("idle state")
            n81 = call-poly <vilib>:"DAQmx Create Virtual Channel.vi"("lines"=tag "Dev1/port1/line0") -> ("task out"=w233:refnum<k21>, "error out"=w236:errorcluster)  [unwired: 13 in]
            n82 = call-poly <vilib>:"DAQmx Write.vi"("task/channels in"=w233, "data"=FALSE, "error in"=w236) -> ("task out"=w235:refnum<k21>, "error out"=w237:errorcluster)  [unwired: 10 in, 1 out]
            n83 = VISA Write(VISA resource name=w239, write buffer="SOUR:SWE:FREQ:MODE AUTO", error in (no error)=w242) -> (VISA resource name out=w249:refnum<visa-resource-name>, error out=w246:errorcluster)  [unwired: 1 out]
            n84 = call-poly <vilib>:"DAQmx Create Virtual Channel.vi"("high ticks"=u32 2, "low ticks"=u32 2, "counter"=tag "Dev1/ctr1", "source of ticks"=tag "/Dev1/100MHzTimebase", "idle state"=w253, "initial delay"=u32 2) -> ("task out"=w262:refnum<k21>)  [unwired: 8 in, 1 out]
            n85 = global read "GLOBAL_VAR.vi" "APD_signal"() -> (w231:tag)
            n86 = call <vilib>:"DAQmx Start Task.vi"("task/channels in"=w235, "error in"=w237) -> ("task out"=w232:refnum<k21>)  [unwired: 12 in, 1 out]
            n87 = call-poly <vilib>:"DAQmx Trigger.vi"("task/channels in"=w262, "source"=w231, "edge"=w257) -> ("task out"=w258:refnum<k21>)  [unwired: 11 in, 1 out]
            n88 = VISA Write(VISA resource name=w249, write buffer="TRIG:FSW:SOUR EXT" ("write buffer 2"), error in (no error)=w246) -> (VISA resource name out=w248:refnum<visa-resource-name>, error out=w247:errorcluster)  [unwired: 1 out]
            n89 = property class="DAQmx Trigger"(reference=w258, "Start.Retriggerable"=TRUE) -> (reference out=w260:refnum<k21>)  [unwired: 1 in, 1 out]
            n90 = VISA Write(VISA resource name=w248, write buffer="SOUR:FREQ:MODE SWE" ("write buffer 3"), error in (no error)=w247) -> (VISA resource name out=w240:refnum<visa-resource-name>, error out=w241:errorcluster)  [unwired: 1 out]
            n91 = call <vilib>:"DAQmx Start Task.vi"("task/channels in"=w260) -> ("task out"=w251:refnum<k21>)  [unwired: 13 in, 1 out]
          }
          frame Error {
            n92 = call <instrlib>:"Reset.vi"("VISA resource name"=w276, "error in (no error)"=w275) -> ("VISA resource name out"=w266:refnum<visa-resource-name>, "error out"=w265:errorcluster)  [unwired: 12 in]
            n93 = call <instrlib>:"Close.vi"("error in (no error)"=w265, "VISA resource name"=w266) -> ("error out"=w271:errorcluster)  [unwired: 9 in]
            n94 = call <vilib>:"Clear Errors.vi"("error in (no error)"=w271, "specific error code to clear (0: all)"=0) -> ("error out"=w264:errorcluster)  [unwired: 4 in, 1 out]
            n95 = Two Button Dialog(message="Erorr: Check connection", 1:"Close" ("F button name (\"Cancel\")"), 2:"Continue" ("T button name (\"OK\")")) -> (T button?=w268:bool)
            n96 = Not(x=w268) -> (.not. x?=w267:bool)
          }
        }
      }
      frame "stand-by", Default {
        n97 = event shown="[2] \"Save\": Value Change" {
          selector: _ -> [_ _ _ _]
          dyn-events: _ -> [_ _ _ _]
          timeout: 10 -> [_ _ _ _]
          tunnel: w292 -> [w310 _ w387 _]
          tunnel: w290 -> [w306 _ w390 _]
          tunnel: w288 -> [w300 w320 w392 w398]
          tunnel: [w300 _ w392 w398] -> w287
          tunnel: [w301 w316 w391 w399] -> w285
          tunnel: w286 -> [w301 w317 w391 w399]
          tunnel: [_ w320 _ _] -> _
          tunnel: w284 -> [_ _ w375 _]
          tunnel: w283 -> [_ _ w372 _]
          tunnel: w282 -> [_ w314 w369 _]
          tunnel: w281 -> [_ _ w364 _]
          tunnel: w280 -> [_ w313 w359 _]
          tunnel: w279 -> [_ _ w342 _]
          tunnel: w278 -> [_ w312 _ _]
          tunnel: [_ w311 _ _] -> w277
          event "Intensity Graph": Cursor Move {
            n98 = event-data() -> ()  [unwired: 1 in, 7 out]
            n99 = property on="Intensity Graph" class="IntGraph (strict)"() -> ("Cursor.Cursor Y"=w308:dbl, "Cursor.Cursor X"=w304:dbl)  [unwired: 2 in, 2 out]
            n100 = Round Toward -Infinity(1:w308) -> (0:w305:dbl)
            n101 = Decrement(x=w305) -> (x-1=w307:dbl)
            n102 = local write "Run"(w305) -> ()
            n103 = Index Array(array=w306, index (row)=w307) -> (element=w309:ext[])  [unwired: 1 in]
            n104 = Bundle(w310, w309) -> (w302:cluster{ext[], ext[]})  [unwired: 1 in]
            n105 = Build Array(w302, w300) -> (w303:cluster{ext[], ext[]}[])
            n106 = local write "Histogram"(w303) -> ()
            n107 = property on="Histogram" class="XYGraph (strict)"("Cursor.Cursor X"=w304) -> ()  [unwired: 2 in, 2 out]
          }
          event "generator_enable": Value Change {
            n108 = event-data() -> ("NewVal"=w315:bool)  [unwired: 1 in, 5 out]
            n109 = call <instrlib>:"Configure RF.vi"("Power Level (-30.0)"=w313, "error in (no error)"=w312, "Frequency (1.0e9)"=w314, "VISA resource name"=w317) -> ("error out"=w319:errorcluster, "VISA resource name out"=w318:refnum<visa-resource-name>)  [unwired: 6 in]
            n110 = call <instrlib>:"Configure Output Enabled.vi"("error in (no error)"=w319, "Output Enabled (Off)"=w315, "VISA resource name"=w318) -> ("error out"=w311:errorcluster, "VISA resource name out"=w316:refnum<visa-resource-name>)  [unwired: 7 in]
          }
          event "Save": Value Change {
            n111 = event-data() -> ()  [unwired: 1 in, 6 out]
            n112 = Number To Fractional String(number=w372, precision (6)=i16 0) -> (F-format string=w373:string)  [unwired: 2 in]
            n113 = Number To Fractional String(number=w369, precision (6)=i16 0) -> (F-format string=w370:string)  [unwired: 2 in]
            n114 = Number To Fractional String(number=w364, precision (6)=i16 3) -> (F-format string=w366:string)  [unwired: 2 in]
            n115 = Number To Fractional String(number=w375, precision (6)=i16 0) -> (F-format string=w376:string)  [unwired: 2 in]
            n116 = Concatenate Strings("Freq start [Hz] = ", w370, "\r\n") -> (w339:string)
            n117 = Concatenate Strings("Dwell time [s] = ", w366, "\r\n") -> (w338:string)
            n118 = Concatenate Strings("Step size [Hz] = ", w376, "\r\n") -> (w341:string)
            n119 = Concatenate Strings("Freq stop [Hz] = ", w373, "\r\n") -> (w340:string)
            n120 = Concatenate Strings(w341, w340, w339, w338) -> (w334:string)
            n121 = Get Date/Time In Seconds() -> (seconds since 1Jan1904=w397:timestamp)
            n122 = Format Date/Time String(time format string (%c)="%Y-%m-%d_%H-%M-%S", seconds (now)=w397) -> (date/time string=w396:string)  [unwired: 1 in]
            n123 = Unbundle("position_xyz") -> ("Position X"=w323:dbl, "Position Y"=w322:dbl, "Position Z"=w321:dbl)
            n124 = Concatenate Strings(w396, ".dsp") -> (w327:string)
            "File name" <- w327
            n125 = Concatenate Strings("D:\\Data\\raw data\\", w327) -> (w325:string)
            n126 = Array To Spreadsheet String(array=w387, 3:"%.0f" ("format string")) -> (spreadsheet string=w386:string)  [unwired: 1 in]
            n127 = Array To Spreadsheet String(array=w390, 3:"%.3f" ("format string")) -> (spreadsheet string=w384:string)  [unwired: 1 in]
            n128 = Number To Fractional String(number=w359, precision (6)=i16 0) -> (F-format string=w361:string)  [unwired: 2 in]
            n129 = Number To Fractional String(number=w323, precision (6)=i16 3) -> (F-format string=w353:string)  [unwired: 2 in]
            n130 = Number To Fractional String(number=w322, precision (6)=i16 3) -> (F-format string=w350:string)  [unwired: 2 in]
            n131 = Number To Fractional String(number=w321, precision (6)=i16 3) -> (F-format string=w344:string)  [unwired: 2 in]
            n132 = String To Path(string=w325) -> (path=w393:path)
            n133 = Number To Fractional String(number=w342, precision (6)=i16 0) -> (F-format string=w358:string)  [unwired: 2 in]
            n134 = Concatenate Strings("Power [dBm] = ", w361, "\r\n") -> (w333:string)
            n135 = Concatenate Strings("Position X [V] = ", w353, "\r\n") -> (w332:string)
            n136 = Concatenate Strings("Position Y [V] = ", w350, "\r\n") -> (w331:string)
            n137 = Concatenate Strings("Position Z [V] = ", w344, "\r\n") -> (w330:string)
            n138 = Concatenate Strings(w386, "\r\n", w384) -> (w336:string)
            n139 = Concatenate Strings("Repetitions = ", w358, "\r\n") -> (w329:string)
            n140 = Concatenate Strings(w334, w333, w332, w331, w330, w329, "\r\n") -> (w335:string)
            n141 = Concatenate Strings(w335, w336) -> (w337:string)
            n142 = call <vilib>:"Write Characters To File.vi"("character string"=w337, "file path (dialog if empty)"=w393) -> ()  [unwired: 3 in, 1 out]
          }
          event Timeout {
            n143 = event-data() -> ()  [unwired: 1 in, 3 out]
          }
        }
        n144 = Not(x="start") -> (.not. x?=w297:bool)
        n145 = Select(t=w299, s=w297, f=T3."Set Variables") -> (s? t:f=w298:T3)
      }
    }
    n146 = Not(x="stop") -> (.not. x?=w33:bool)
    n147 = Select(t=w31, s=w33, f=T3."close") -> (s? t:f=w30:T3)
  }
